vi "Launch Nested Actor.vi"(6 "Auto Stop?":bool, 8 "error in (no error)":errorcluster, 9 "Actor Name":string, 10 "Nested Mediated Asynchronous Actor in":refnum<class "Mediated Asynchronous Actor.lvclass">, 11 "Caller Mediated Asynchronous Actor in":refnum<class "Mediated Asynchronous Actor.lvclass">) -> (0 "error out":errorcluster, 2 "Nested Mediated Asynchronous Actor's Message Transport":refnum<class "Message Transport Interface.lvclass">, 3 "Caller Mediated Asynchronous Actor out":refnum<class "Mediated Asynchronous Actor.lvclass">)   [LabVIEW 2016, in "Stream Mediator.lvlib" / "Mediated Asynchronous Actor.lvclass"]
doc: "--\nCopyright © 2017 Composed SystemsI All rights reserved.\n\nAuthor: Jon McBee <jon.mcbee@composed.io>\n\nThis library is provided \"AS IS\" ,WITHOUT WARRANTIES OR\nCONDITIONS OF ANY KIND, either express or implied.\n\nComposed Systems -- composed.io\n\nStream 0.0.1.1\nJon McBee - Composed Systems\nCopyright (c) 2017, Composed Systems"
uses:
  <userlib>/Composed Systems/Stream/Mediator/Classes/Mediated Asynchronous Actor/Mediated Asynchronous Actor.lvclass
  C:/Program Files (x86)/National Instruments/LabVIEW 2016/user.lib/Composed Systems/Stream/Mediator/Classes/Mediated Actor/Mediated Actor.lvclass
  <userlib>/Composed Systems/Stream/Mediator/Classes/Message Transport Interface/Message Transport Interface.lvclass
  <userlib>/Composed Systems/Stream/Mediator/Classes/Mediated Actor/Mediated Actor.lvclass
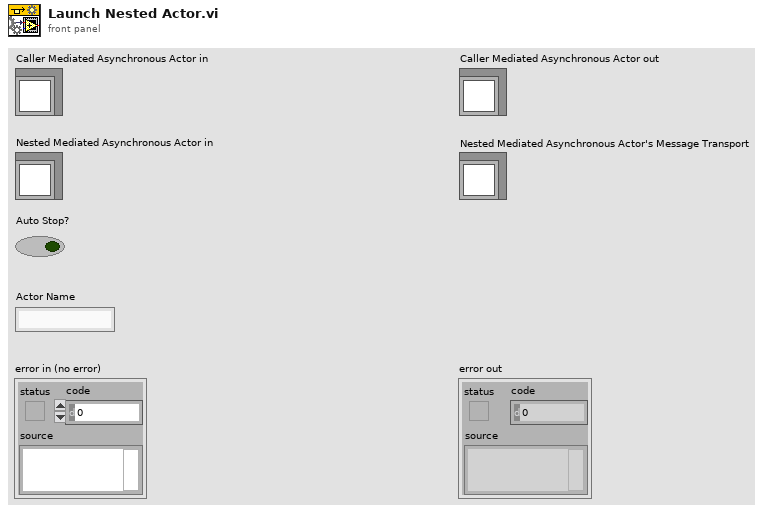
[diagram p1: front panel]
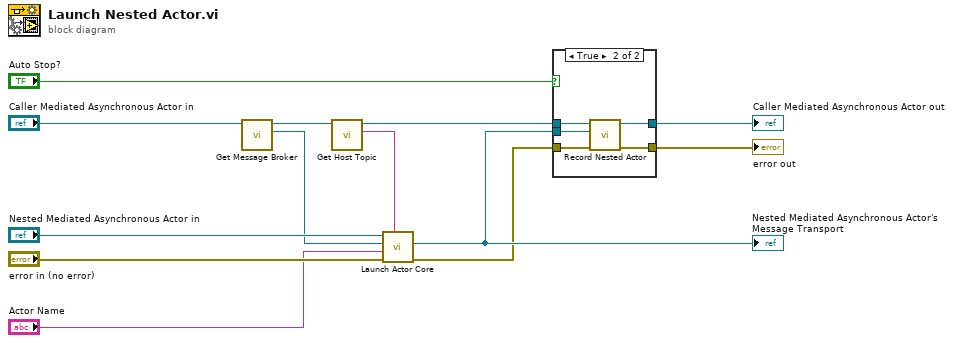
[diagram p0: block diagram]
diagram:
  n1 = call <userlib>:"Get Message Broker.vi"("Mediated Actor in"="Caller Mediated Asynchronous Actor in") -> ("Message Broker"=w8:refnum<class "Message Broker Interface.lvclass">, "Mediated Actor out"=w12:refnum<class "Mediated Asynchronous Actor.lvclass">)  [unwired: 9 in]
  n2 = call <userlib>:"Get Host Topic.vi"("Mediated Actor in"=w12) -> ("Topic.Host"=w9:string, "Mediated Actor out"=w6:refnum<class "Mediated Asynchronous Actor.lvclass">)  [unwired: 9 in]
  n3 = call <userlib>:"Launch Actor Core.vi"("Host Name"=w9, "error in (no error)"="error in (no error)", "Actor Name"="Actor Name", "Message Broker"=w8, "Mediated Asynchronous Actor in"="Nested Mediated Asynchronous Actor in") -> ("error out"=w3:errorcluster, "Message Transport"=w4:refnum<class "Message Transport Interface.lvclass">)  [unwired: 5 in]
  "Nested Mediated Asynchronous Actor's Message Transport" <- w4
  n4 = case shown="True" "Auto Stop?" {
    tunnel: w6 -> [w15 w20]
    tunnel: [w15 w19] -> w5
    tunnel: w4 -> [_ w18]
    tunnel: w3 -> [w14 w17]
    tunnel: [w14 w16] -> w2
    frame False {
    }
    frame True {
      n5 = call <userlib>:"Record Nested Actor.vi"("error in (no error)"=w17, "Nested Mediated Asynchronous Actor's Message Transport"=w18, "Mediated Asynchronous Actor in"=w20) -> ("error out"=w16:errorcluster, "Mediated Asynchronous Actor out"=w19:refnum<class "Mediated Asynchronous Actor.lvclass">)  [unwired: 7 in]
    }
  }
  "error out" <- w2
  "Caller Mediated Asynchronous Actor out" <- w5
